vi "Write Exporter parameters.vi"(9 "Parameters":string, 11 "UIManager in":refnum<class "UIManager.lvclass">) -> (3 "UIManager out":refnum<class "UIManager.lvclass">)   [LabVIEW 2020, in "DependencyInspector.lvlib" / "UIManager.lvclass"]
uses:
  UIManager.lvclass
  UIManager.lvclass/UIManager.ctl
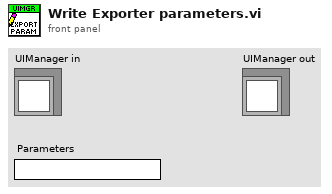
[diagram p1: front panel]
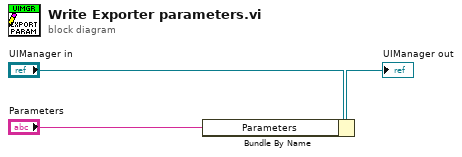
[diagram p0: block diagram]
diagram:
  n1 = Bundle By Name(cluster="UIManager in", "Parameters"="Parameters") -> (→"UIManager out":refnum<class "UIManager.lvclass">)
